vi "Disabled.vi"(7 "Robot Mode":T2, 10 "Match Info":T1={"Autonomous Elapsed Seconds"=0.0, "TeleOp Elapsed Seconds"=0.0, "Disabled Elapsed Seconds"=0.0, "Visited Autonomous"=FALSE, "Visited TeleOp"=FALSE, "Visited Disabled"=FALSE, "Autonomous Settings"={"Autonomous Style"=enum."Independent", "VI Refnum"=refnum}}, 11 "Call Context":T3) -> ()   [LabVIEW 2016]
doc: "This VI is called each time a disabled packet is received from the DS. It is often used to prepare for the next robot mode, to calibrate sensors, etc."
uses:
  <vilib>/Rock Robotics/WPI/DriverStation/WPI_DriverStationDerivedRobotMode.ctl
  <vilib>/Rock Robotics/WPI/DriverStation/WPI_DriverStationRobotMode2.ctl
  <vilib>/Rock Robotics/WPI/DriverStation/WPI_DriverStationMatch Info.ctl
  Autonomous VIs/Robot Subsystems.ctl
  Drive/Drive Notifier.ctl
  Drive/Drive Control Type.ctl
  Climb/Climb Notifier.ctl
  Climb/Climb Control Type.ctl
  Intake/Intake Notifier.ctl
  Intake/Intake Control Type.ctl
  Rotation/Rotation Notifier.ctl
  Rotation/Rotation Control Type.ctl
  Autonomous VIs/Queue Key Data.ctl
  <vilib>/Rock Robotics/Network Tables/NT Write String.vi
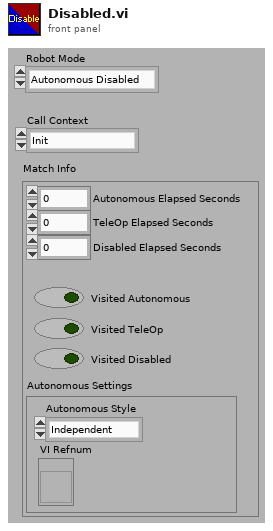
[diagram p1: front panel]
types:
  T1 = typedef "WPI_DriverStationMatch Info.ctl" = cluster{"Autonomous Elapsed Seconds":dbl, "TeleOp Elapsed Seconds":dbl, "Disabled Elapsed Seconds":dbl, "Visited Autonomous":bool, "Visited TeleOp":bool, "Visited Disabled":bool, "Autonomous Settings":cluster{"Autonomous Style":enum16{"Iterative", "Independent"}, "VI Refnum":refnum<vi>}}
  T2 = typedef "WPI_DriverStationRobotMode2.ctl" = enum16{"Autonomous Disabled", "Autonomous Enabled", "Teleop Disabled", "Teleop Enabled", "Disconnected", "Finish", "Test Disabled", "Test Enabled", "Emergency Stopped"}
  T3 = typedef "WPI_DriverStationDerivedRobotMode.ctl" = enum16{"Init", "Execute", "Stop"}
  T4 = typedef "Queue Key Data.ctl" = cluster{"Operation Notifier":refnum<notifier>, "Subsystem":string, "Concurrent":bool}
  T5 = typedef "Robot Subsystems.ctl" = cluster{"Drive Notifier":T6, "Climb Notifier":T8, "Intake Notifier":T10, "Rotation Notifier":T12}
  T6 = typedef "Drive Notifier.ctl" = cluster{"Parameter 1":dbl, "Parameter 2":dbl, "Parameter 3":dbl, "Drive Control List":T7, "Parameter 4":dbl, "Gear Angle":dbl, "Parameter 6":dbl, "Parameter 7":dbl, "Parameter 8":dbl, "Parameter 9":dbl, "Robotcentric":bool, "Reset Gyro":bool, "Reset Wheels":bool, "Turn to Gear Left":bool, "Turn to Gear Center":bool, "Turn to Gear Right":bool, "Half Power":bool, "Drive Notifier":refnum<notifier>, "Step":i32}
  T7 = typedef "Drive Control Type.ctl" = enum16{"No Op", "Fieldcentric", "Robotcentric", "Reset Wheel Position", "Reset Gyro Value", "Turn to Angle", "Drive For Time"}
  T8 = typedef "Climb Notifier.ctl" = cluster{"Up":bool, "Down":bool, "Climb Control List":T9}
  T9 = typedef "Climb Control Type.ctl" = enum16{"No Op", "Up", "Down"}
  T10 = typedef "Intake Notifier.ctl" = cluster{"In":bool, "Out":bool, "Intake Control List":T11, "Parameter 1":dbl, "Parameter 2":dbl, "Intake Notifier":refnum<notifier>, "Step":i32}
  T11 = typedef "Intake Control Type.ctl" = enum16{"No Op", "In", "Out"}
  T12 = typedef "Rotation Notifier.ctl" = cluster{"Up":bool, "Down":bool, "Rotation Control List":T13, "Control Down":bool, "Manual":bool, "Parameter 1":dbl, "Parameter 2":dbl, "Rotation Notifier":refnum<notifier>, "Step":i32}
  T13 = typedef "Rotation Control Type.ctl" = enum16{"No Op", "Up", "Down", "Control Up", "Control Down"}
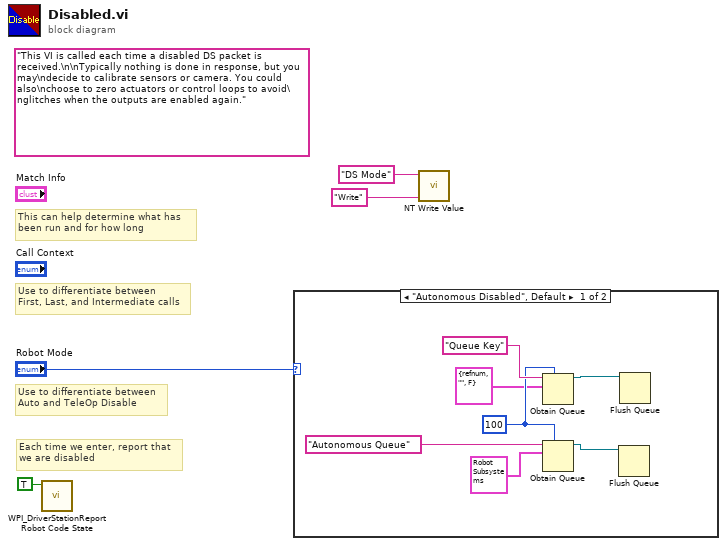
[diagram p0: block diagram]
diagram:
  (unwired) "This VI is called each time a disabled DS packet is received.\n\nTypically nothing is done in response, but you may\ndecide to calibrate sensors or camera. You could also\nchoose to zero actuators or control loops to avoid\nglitches when the outputs are enabled again."
  # "Each time we enter, report that\nwe are disabled"
  # "Use to differentiate between\nFirst, Last, and Intermediate calls"
  # "This can help determine what has\nbeen run and for how long"
  # "Use to differentiate between\nAuto and TeleOp Disable"
  n1 = call <vilib>:"WPI_DriverStationReport Robot Code State.vi"("Disabled"=TRUE ("Autonomous")) -> ()  [unwired: 10 in, 1 out]
  n2 = case shown="\"Autonomous Disabled\", Default" "Robot Mode" {
    frame "Autonomous Disabled", Default {
      w6 = 100 ("max queue size (-1, unlimited)")
      n3 = Obtain Queue(max queue size (-1, unlimited)=w6, name (unnamed)="Queue Key", element data type=T4 {"Operation Notifier"=refnum, "Subsystem"="", "Concurrent"=FALSE} ("Queue Key Data")) -> (queue out=w8:refnum<queue>)  [unwired: 2 in, 2 out]
      n4 = Obtain Queue(max queue size (-1, unlimited)=w6, name (unnamed)="Autonomous Queue", element data type=T5 {"Drive Notifier"={"Parameter 1"=0.0, "Parameter 2"=0.0, "Parameter 3"=0.0, "Drive Control List"=enum."No Op", "Parameter 4"=0.0, "Gear Angle"=0.0, "Parameter 6"=0.0, "Parameter 7"=0.0, "Parameter 8"=0.0, "Parameter 9"=0.0, "Robotcentric"=FALSE, "Reset Gyro"=FALSE, "Reset Wheels"=FALSE, "Turn to Gear Left"=FALSE, "Turn to Gear Center"=FALSE, "Turn to Gear Right"=FALSE, "Half Power"=FALSE, "Drive Notifier"=refnum, "Step"=0}, "Climb Notifier"={"Up"=FALSE, "Down"=FALSE, "Climb Control List"=enum."No Op"}, "Intake Notifier"={"In"=FALSE, "Out"=FALSE, "Intake Control List"=enum."No Op", "Parameter 1"=0.0, "Parameter 2"=0.0, "Intake Notifier"=refnum, "Step"=0}, "Rotation Notifier"={"Up"=FALSE, "Down"=FALSE, "Rotation Control List"=enum."No Op", "Control Down"=FALSE, "Manual"=FALSE, "Parameter 1"=0.0, "Parameter 2"=0.0, "Rotation Notifier"=refnum, "Step"=0}} ("Robot Subsytems")) -> (queue out=w7:refnum<queue>)  [unwired: 2 in, 2 out]
      n5 = Flush Queue(queue=w7) -> ()  [unwired: 1 in, 3 out]
      n6 = Flush Queue(queue=w8) -> ()  [unwired: 1 in, 3 out]
    }
    frame "Autonomous Enabled" {
    }
  }
  n7 = call-poly <vilib>:"NT Write Value.vi"("String"="Write", "Name"="DS Mode") -> ()  [unwired: 9 in, 1 out]
